vi "Bundle.vi"(6 "Sample Interval (-1s)":dbl=-1.0 format="%.2f", 7 "Trigger Type Index(0)":u16, 8 "error in (no error)":errorcluster, 9 "Samples per Trigger(1)":i32=1, 10 "Triggers to measure(1)":i32=1, 11 "DMM Config Trigger Msg in":refnum<class "DMM Config Trigger Msg.lvclass">) -> (0 "error out":errorcluster, 3 "DMM Config Trigger Msg out":refnum<class "DMM Config Trigger Msg.lvclass">)   [LabVIEW 2020, in "DMM Msg.lvlib" / "DMM Config Trigger Msg.lvclass"]
doc: "Populate the message data."
uses:
  DMM Config Trigger Msg.lvclass
  DMM Config Trigger Msg.lvclass/DMM Config Trigger Msg.ctl
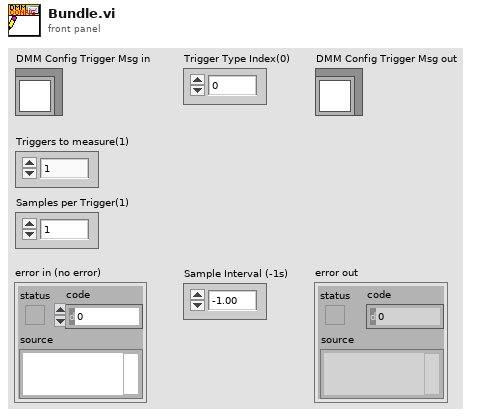
[diagram p1: front panel]
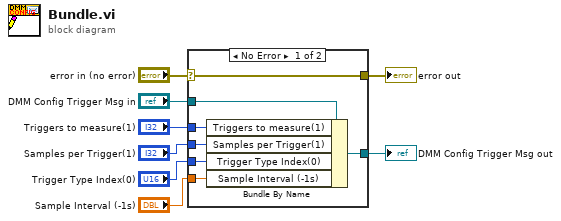
[diagram p0: block diagram]
diagram:
  n1 = case shown="No Error" "error in (no error)" {
    selector: "error in (no error)" -> [w15 w16]
    tunnel: [w15 w16] -> w7
    tunnel: [w13 w17] -> w5
    tunnel: "DMM Config Trigger Msg in" -> [w14 w17]
    tunnel: "Triggers to measure(1)" -> [w12 _]
    tunnel: "Trigger Type Index(0)" -> [w11 _]
    tunnel: "Sample Interval (-1s)" -> [w10 _]
    tunnel: "Samples per Trigger(1)" -> [w9 _]
    frame No Error {
      n2 = Bundle By Name(cluster=w14, "Triggers to measure(1)"=w12, "Samples per Trigger(1)"=w9, "Trigger Type Index(0)"=w11, "Sample Interval (-1s)"=w10) -> (w13:refnum<class "DMM Config Trigger Msg.lvclass">)
    }
    frame Error {
    }
  }
  "error out" <- w7
  "DMM Config Trigger Msg out" <- w5
